vi "Initialize Front Panel.vi"(8 "error in (no error)":errorcluster, 11 "GarphView in":refnum<class "GarphView.lvclass">) -> (0 "error out":errorcluster, 3 "GarphView out":refnum<class "GarphView.lvclass">)   [LabVIEW 2020, in "GarphView.lvlib" / "GarphView.lvclass"]
doc: "<License>\nCopyright © 2017 Composed Systems, LLC | All rights reserved\nwww.composed.io\n\nAuthor: Ethan Stern <ethan.stern@composed.io>\n\nThis software is provided \"AS IS\" WITHOUT WARRANTIES, either express or implied, AND IS FOR EDUCATIONAL PURPOSES ONLY.\n</License>"
uses:
  GarphView.lvclass
  GarphView.lvclass/GarphView.ctl
  <vilib>/gpm_packages/@cs/mva-viewable/Source/IViewable/IViewable/IViewable.lvclass
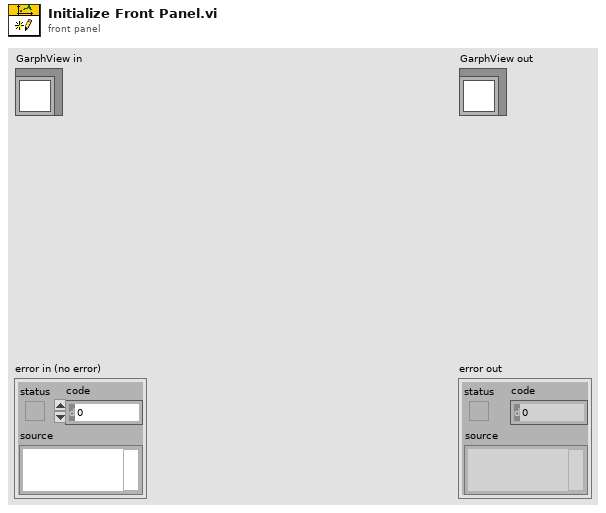
[diagram p1: front panel]
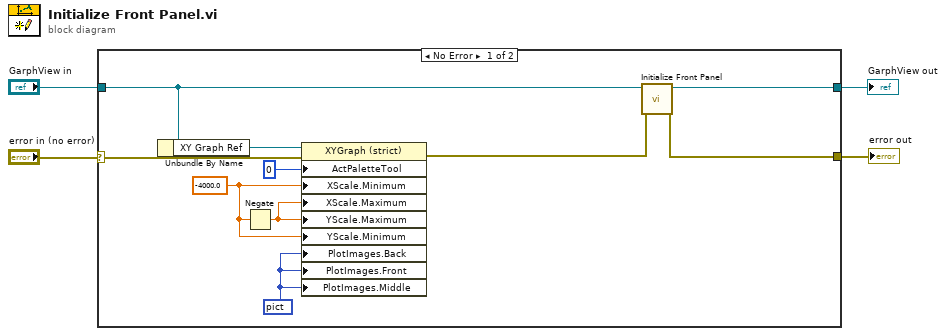
[diagram p0: block diagram]
diagram:
  n1 = case shown="No Error" "error in (no error)" {
    selector: "error in (no error)" -> [w6 w16]
    tunnel: [w14 w16] -> w4
    tunnel: [w13 w15] -> w3
    tunnel: "GarphView in" -> [w11 w15]
    frame No Error {
      w5 = picture data[5B] ("Plot Images:Back")
      w8 = -4000.0 ("X Scale.Range:Minimum")
      n2 = Unbundle By Name(w11) -> ("XY Graph Ref"=w10:refnum<vi>)
      n3 = Negate(x=w8) -> (-x=w9:dbl)
      n4 = property on="Property Node" class="XYGraph (strict)"(reference=w10, error in=w6, "ActPaletteTool"=0 ("Palette:Active Tool"), "XScale.Minimum"=w8, "XScale.Maximum"=w9, "YScale.Maximum"=w9, "YScale.Minimum"=w8, "PlotImages.Back"=w5, "PlotImages.Front"=w5, "PlotImages.Middle"=w5) -> (error out=w7:errorcluster)  [unwired: 1 out]
      n5 = call-parent "Initialize Front Panel.vi"("error in (no error)"=w7, "IViewable in"=w11) -> ("error out"=w14:errorcluster, "IViewable out"=w13:refnum<class "GarphView.lvclass">)  [unwired: 8 in]
    }
    frame Error {
    }
  }
  "error out" <- w4
  "GarphView out" <- w3
